vi "Get REF StringsAndValues.vi"(8 "error in (no error)":errorcluster, 11 "Instrument.Lockin in":refnum<class "Instrument.Lockin.lvclass">) -> (0 "error out":errorcluster, 2 "REF Strings and Values":cluster{string, i32}[](array[cluster]), 3 "Instrument.Lockin out":refnum<class "Instrument.Lockin.lvclass">)   [LabVIEW 2016, in "Instrument.Lockin.lvclass"]
uses:
  Instrument.Lockin.lvclass
  Instrument.Lockin.lvclass/Instrument.Lockin.ctl
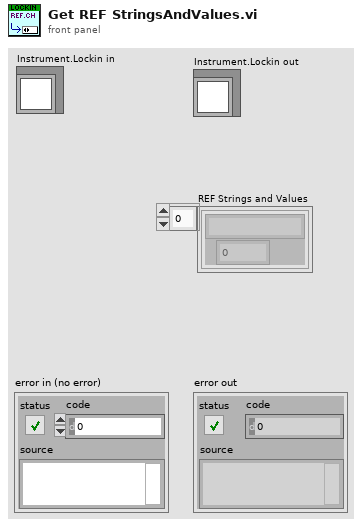
[diagram p1: front panel]
types:
  T1 = typedef "Lockin.DAQ.lvclass/REF-cluster.ctl" = T2[]
  T2 = typedef "Instrument.Lockin.UI.lvclass/REF Channel--Cluster.ctl" = cluster{"Enable?":bool, "Channel":i32, "Frequency":dbl, "Phase":dbl, "TC":dbl, "Order":i32}
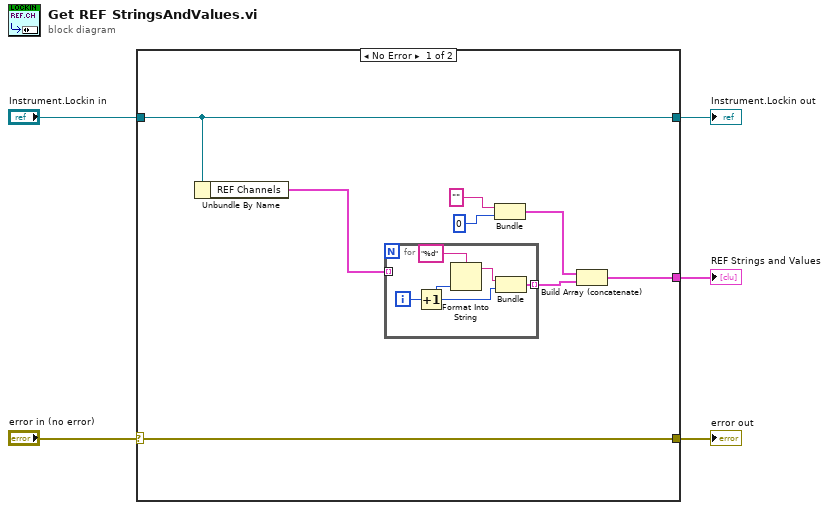
[diagram p0: block diagram]
diagram:
  n1 = case shown="No Error" "error in (no error)" {
    selector: "error in (no error)" -> [w12 w20]
    tunnel: "Instrument.Lockin in" -> [w13 w19]
    tunnel: [w7 _] -> w4
    tunnel: [w13 w19] -> w2
    tunnel: [w12 w20] -> w1
    frame No Error {
      n2 = Unbundle By Name(w13) -> ("REF Channels"=w11:T1)
      n3 = for {
        tunnel: [w17] -> w6 mode=indexing
        tunnel: w11 -> [_] mode=indexing
        i -> [w18]
        n4 = Increment(x=w18) -> (x+1=w16:i32)
        n5 = Format Into String(format string="%d", w16) -> (resulting string=w14:string)  [unwired: 2 in, 1 out]
        n6 = Bundle(w14, w16) -> (w17:cluster{string, i32})  [unwired: 1 in]
      }
      n7 = Bundle("format string"="", "x+1"=0) -> (w8:cluster{"format string":string, "x+1":i32})  [unwired: 1 in]
      n8 = Build Array (concatenate)(w8, w6) -> (w7:cluster{"format string":string, "x+1":i32}[])
    }
    frame Error {
    }
  }
  "REF Strings and Values" <- w4
  "Instrument.Lockin out" <- w2
  "error out" <- w1
